vi "delete indexes from array.vi"(1 "indexes removed":i32[](array[numeric]), 2 "array in":dbl[](array[numeric])) -> (0 "array out":dbl[](array[numeric]))   [LabVIEW 2009]
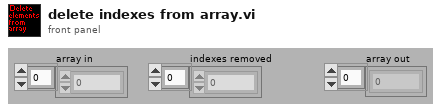
[diagram p1: front panel]
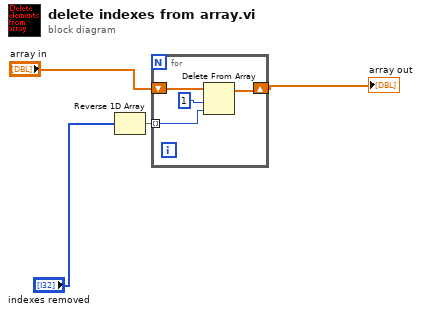
[diagram p0: block diagram]
diagram:
  n1 = Reverse 1D Array(array="indexes removed") -> (reversed array=w1:i32[])
  n2 = for {
    tunnel: w1 -> [w8] mode=indexing
    shift-right: [w6] -> w4
    shift-left: "array in" -> [w7]
    n3 = Delete From Array(array=w7, length=1, index=w8) -> (array with subset deleted=w6:dbl[])  [unwired: 1 out]
  }
  "array out" <- w4
